vi "ma_SML Spectrum Peak Search (basic).vi"(8 "error in (no error)":errorcluster, 9 "peak search settings":T2 {"Threshold" format="%.2f"}, 10 "spectral info":T1 {"window" items=["Rectangle"=0, "Hanning"=1, "Hamming"=2, "Blackman-Harris"=3, "Exact Blackman"=4, "Blackman"=5, "Flat Top"=6, "4 Term B-Harris "=7, "7 Term B-Harris"=8, "Low Sidelobe"=9, "Blackman Nuttall"=11, "Triangle"=30, "Bartlett-Hanning"=31, "Bohman"=32, "Parzen"=33, "Welch"=34, "Kaiser"=60, "Dolph-Chebyshev"=61, "Gaussian"=62]}, 11 "spectrum":T3={"f0"=1.0, "df"=1.0, "spectrum"=[]} {"spectrum" format="%.2f"; "df" format="%.2f"; "f0" format="%.2f"}) -> (0 "error out":errorcluster, 2 "# of peaks":i32, 3 "peaks":cluster{"frequency":dbl, "Value":dbl}[](array[cluster]) {"Value" format="%.2f"; "frequency" format="%.2f"})   [LabVIEW 2020, in "NI_MAPro.lvlib"]
uses:
  NI_MAPro.lvlib
  ma_sml_Spectrum Cluster (real).ctl
  ma_sml_Spectral Info.ctl
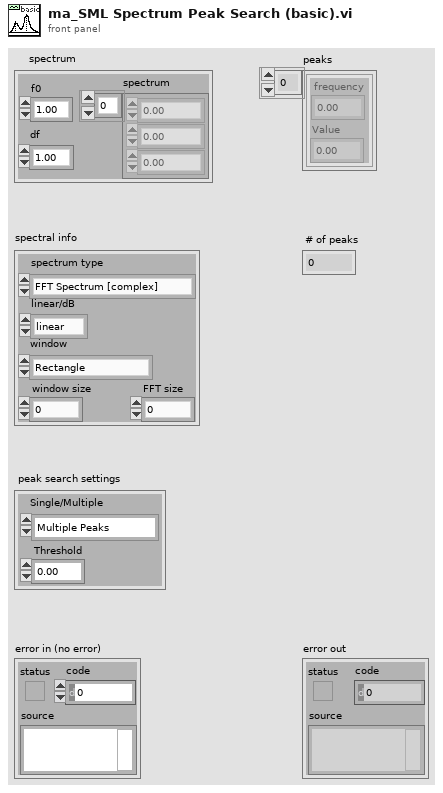
[diagram p1: front panel]
types:
  T1 = typedef "NI_MAPro.lvlib/ma_sml_Spectral Info.ctl" = cluster{"spectrum type":enum16{"FFT Spectrum [complex]", "Amplitude [Magnitude]", "Power [Magnitude^2]", "Cross Spectrum [complex]", "Frequency Response [Complex]"}, "linear/dB":enum16{"linear", "dB"}, "window":u16, "window size":i32, "FFT size":i32}
  T2 = cluster{"Single/Multiple":enum16{"Multiple Peaks", "Single Max Peak"}, "Threshold":dbl}
  T3 = typedef "NI_MAPro.lvlib/ma_sml_Spectrum Cluster (real).ctl" = cluster{"f0":dbl, "df":dbl, "spectrum":dbl[]}
  T4 = enum16{"FFT Spectrum [complex]", "Amplitude [Magnitude]", "Power [Magnitude^2]", "Cross Spectrum [complex]", "Frequency Response [Complex]"}
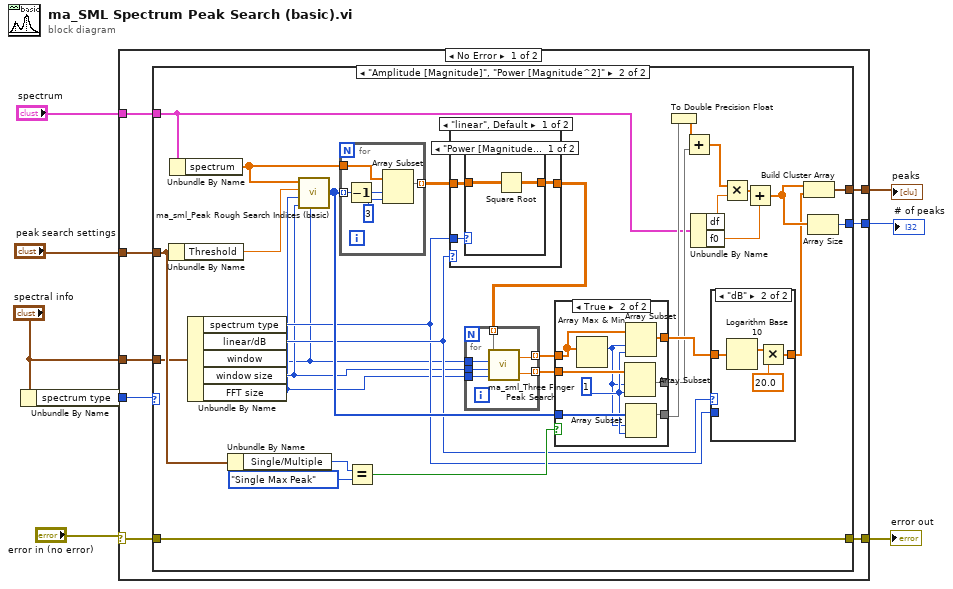
[diagram p0: block diagram]
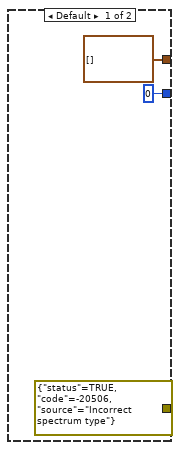
[diagram p2: hidden frame]
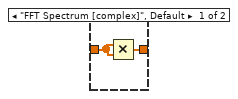
[diagram p4: hidden frame]
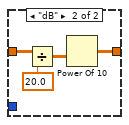
[diagram p7: hidden frame]
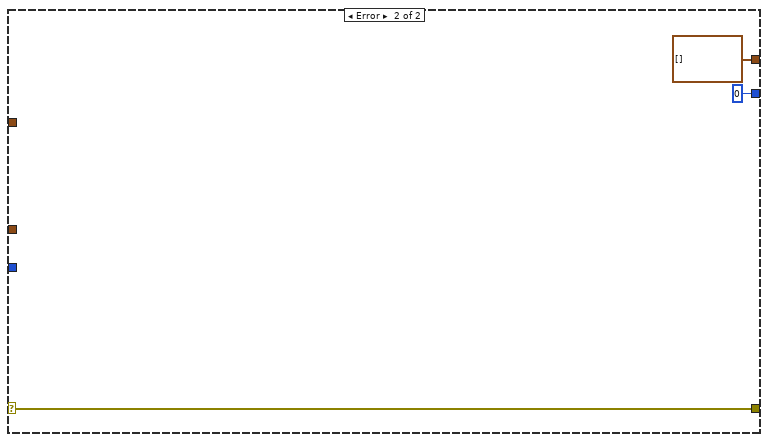
[diagram p8: hidden frame]
diagram:
  n1 = Unbundle By Name("spectral info") -> ("spectrum type"=w5:T4)
  n2 = case shown="No Error" "error in (no error)" {
    selector: "error in (no error)" -> [w14 w95]
    tunnel: "spectral info" -> [w16 _]
    tunnel: [w13 w95] -> w7
    tunnel: w5 -> [w15 _]
    tunnel: [w12 cluster{dbl, "amplitude":dbl}[] []] -> w4
    tunnel: [w11 0] -> w3
    tunnel: "peak search settings" -> [w10 _]
    tunnel: "spectrum" -> [w9 _]
    frame No Error {
      n3 = case shown="\"Amplitude [Magnitude]\", \"Power [Magnitude^2]\"" w15 {
        tunnel: w16 -> [_ w28]
        tunnel: w14 -> [_ w23]
        tunnel: [errorcluster {"status"=TRUE, "code"=-20506, "source"="Incorrect spectrum type"} ("error IO") w23] -> w13
        tunnel: [cluster{dbl, "amplitude":dbl}[] [] w22] -> w12
        tunnel: [0 w21] -> w11
        tunnel: w10 -> [_ w46]
        tunnel: w9 -> [_ w20]
        frame Default {
        }
        frame "Amplitude [Magnitude]", "Power [Magnitude^2]" {
          n4 = Unbundle By Name(w46) -> ("Threshold"=w31:dbl)
          n5 = Unbundle By Name(w20) -> ("spectrum"=w30:dbl[])
          n6 = Unbundle By Name(w28) -> ("spectrum type"=w34:T4, "linear/dB"=w35:enum16{"linear", "dB"}, "window"=w29:u16, "window size"=w33:i32, "FFT size"=w32:i32)
          n7 = Unbundle By Name(w46) -> ("Single/Multiple"=w44:enum16{"Multiple Peaks", "Single Max Peak"})
          n8 = call "ma_sml_Peak Rough Search Indices (basic).vi"("x"=w30, "threshold"=w31, "FFT Size"=w32, "Window Size"=w33, "window"=w29) -> ("peak indice"=w37:i32[])
          n9 = for {
            tunnel: w37 -> [w88] mode=indexing
            tunnel: w30 -> [w92]
            tunnel: [w89] -> w47 mode=indexing
            n10 = Decrement(x=w88) -> (x-1=w90:i32)
            n11 = Array Subset(array=w92, index=w90, length=3 ("Array Length")) -> (w89:dbl[])
          }
          n12 = Equal?(x=w44, y=enum16{"Multiple Peaks", "Single Max Peak"}."Single Max Peak" ("Output Element")) -> (x = y?=w42:bool)
          n13 = case shown="\"linear\", Default" w35 {
            tunnel: w47 -> [w80 w87]
            tunnel: [w79 w86] -> w45
            tunnel: w34 -> [w78 _]
            frame "linear", Default {
              n14 = case shown="\"Power [Magnitude^2]\", Default" w78 {
                tunnel: w80 -> [w82 w83]
                tunnel: [w81 w83] -> w79
                frame "Power [Magnitude^2]", Default {
                  n15 = Square Root(x=w82) -> (sqrt(x)=w81:dbl[][])
                }
                frame "Amplitude [Magnitude]" {
                }
              }
            }
            frame "dB" {
              n16 = Divide(x=w87, y=20.0 ("x")) -> (x/y=w84:dbl[][])
              n17 = Power Of 10(x=w84) -> (10^x=w86:dbl[][])
            }
          }
          n18 = for {
            tunnel: [w77] -> w41 mode=indexing
            tunnel: [w76] -> w40 mode=indexing
            tunnel: w45 -> [w75] mode=indexing
            tunnel: w29 -> [w74]
            tunnel: w33 -> [w73]
            tunnel: w32 -> [w72]
            n19 = call "ma_sml_Three Finger Peak Search.vi"("FFT Size"=w72, "window length"=w73, "window"=w74, "three fingers"=w75) -> ("freq"=w76:dbl, "amplitude"=w77:dbl)
          }
          n20 = case shown="True" w42 {
            tunnel: w41 -> [w63 w71]
            tunnel: [w63 w68] -> w39
            tunnel: w40 -> [w62 w70]
            tunnel: [w62 w69] -> w25
            tunnel: w37 -> [w61 w67]
            tunnel: [w61 w64] -> w36
            frame False {
            }
            frame True {
              w66 = 1 ("Array Length")
              n21 = Array Max & Min(array=w71) -> (max index (indices)=w65:i32)  [unwired: 3 out]
              n22 = Array Subset(array=w70, index=w65, length=w66) -> (w69:dbl[])
              n23 = Array Subset(array=w71, index=w65, length=w66) -> (w68:dbl[])
              n24 = Array Subset(array=w67, index=w65, length=w66) -> (w64:i32[])
            }
          }
          n25 = To Double Precision Float(number=w36) -> (double precision float=w24:dbl[])
          n26 = Add(x=w24, y=w25) -> (x+y=w38:dbl[])
          n27 = Unbundle By Name(w20) -> ("df"=w49:dbl, "f0"=w48:dbl)
          n28 = case shown="\"dB\"" w35 {
            tunnel: w39 -> [w53 w60]
            tunnel: [w52 w59] -> w26
            tunnel: w34 -> [w51 _]
            frame "linear", Default {
              n29 = case shown="\"Amplitude [Magnitude]\"" w51 {
                tunnel: w53 -> [w54 w56]
                tunnel: [w55 w56] -> w52
                frame "FFT Spectrum [complex]", Default {
                  n30 = Multiply(x=w54, y=w54) -> (x*y=w55:dbl[])
                }
                frame "Amplitude [Magnitude]" {
                }
              }
            }
            frame "dB" {
              n31 = Logarithm Base 10(1:w60) -> (0:w57:dbl[])
              n32 = Multiply(x=w57, y=20.0 ("x")) -> (x*y=w59:dbl[])
            }
          }
          n33 = Multiply(x=w38, y=w49) -> (x*y=w50:dbl[])
          n34 = Add(x=w50, y=w48) -> (x+y=w27:dbl[])
          n35 = Build Cluster Array(w27, w26) -> (w22:cluster{dbl, "amplitude":dbl}[])
          n36 = Array Size(array=w27) -> (size(s)=w21:i32)
        }
      }
    }
    frame Error {
    }
  }
  "error out" <- w7
  "peaks" <- w4
  "# of peaks" <- w3
